vi "Write LabVIEW Version to LVPROJ File.vi"(8 "error in":errorcluster, 10 "LabVIEW Version":string, 11 "Project File Path":path) -> (0 "error out":errorcluster, 2 "Previous Version":string)   [LabVIEW 2020, in "Save for Previous Version.lvlib" / "LabVIEW Project File.lvclass"]
uses:
  LabVIEW Project File.lvclass
  LabVIEW Project File.lvclass/LabVIEW Project File.ctl
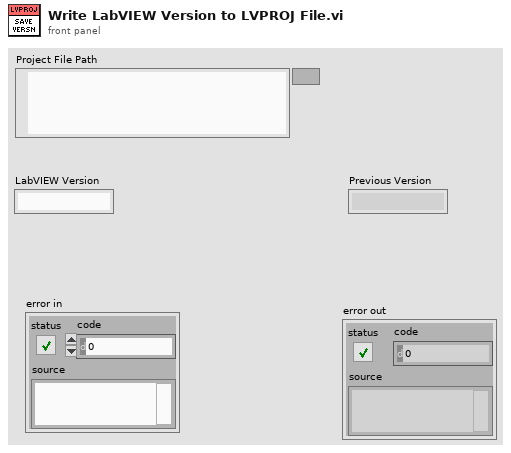
[diagram p1: front panel]
types:
  T1 = enum16{"open", "replace", "create", "open or create", "replace or create", "replace or create with confirmation"}
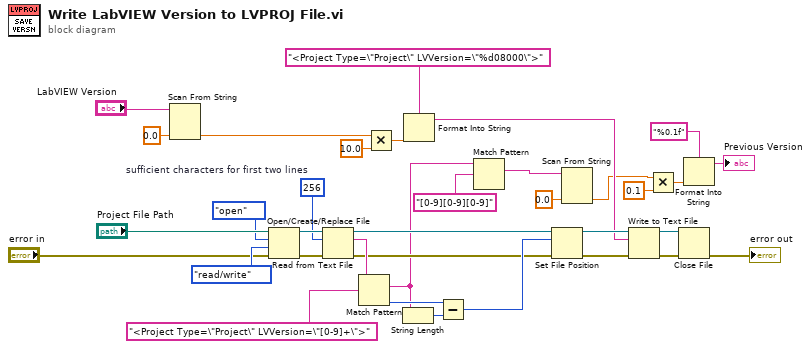
[diagram p0: block diagram]
diagram:
  w1 = 256  # sufficient characters for first two lines
  n1 = Scan From String(input string="LabVIEW Version", default 1=0.0 ("default value 1")) -> (output 1=w30:dbl)  [unwired: 3 in, 3 out]
  n2 = Open/Create/Replace File(file path (use dialog)="Project File Path", error in="error in", operation (0:open)=T1."open", access (0:read/write)=enum16{"read/write", "read-only", "write-only"}."read/write") -> (refnum out=w17:refnum<file>, error out=w15:errorcluster)  [unwired: 2 in, 1 out]
  n3 = Read from Text File(file (use dialog)=w17, count=w1, error in=w15) -> (refnum out=w25:refnum<file>, text=w34:string, error out=w23:errorcluster)  [unwired: 1 in, 1 out]
  n4 = Match Pattern(string=w34, regular expression="<Project Type=\"Project\" LVVersion=\"[0-9]+\">") -> (match substring=w11:string, offset past match=w27:i32)  [unwired: 1 in, 2 out]
  n5 = Multiply(x=w30, y=10.0 ("default value 1")) -> (x*y=w29:dbl)
  n6 = String Length(string=w11) -> (length=w26:i32)
  n7 = Format Into String(format string="<Project Type=\"Project\" LVVersion=\"%d08000\">" ("regular expression"), w29) -> (resulting string=w20:string)  [unwired: 2 in, 1 out]
  n8 = Subtract(x=w27, y=w26) -> (x-y=w24:i32)
  n9 = Match Pattern(string=w11, regular expression="[0-9][0-9][0-9]") -> (match substring=w8:string)  [unwired: 1 in, 3 out]
  n10 = Set File Position(offset (in bytes) (0)=w24, refnum=w25, error in=w23) -> (refnum out=w21:refnum<file>, error out=w22:errorcluster)  [unwired: 1 in]
  n11 = Scan From String(input string=w8, default 1=0.0 ("default value 1")) -> (output 1=w6:dbl)  [unwired: 3 in, 3 out]
  n12 = Write to Text File(file (use dialog)=w21, text=w20, error in=w22) -> (refnum out=w18:refnum<file>, error out=w19:errorcluster)  [unwired: 1 in, 1 out]
  n13 = Multiply(x=w6, y=0.1 ("default value 1")) -> (x*y=w5:dbl)
  n14 = Close File(refnum=w18, error in=w19) -> (error out=→"error out":errorcluster)  [unwired: 1 out]
  n15 = Format Into String(format string="%0.1f", w5) -> (resulting string=→"Previous Version":string)  [unwired: 2 in, 1 out]
